vi "make magnet graph from elements.vi"(7 "mag type":enum16{"absolute", "relative", "positional"}(ring), 10 "toffset":dbl, 11 "elements":T2[](array[typedef])) -> (2 "t offset out":dbl, 3 "graphs":T1)   [LabVIEW 2017]
uses:
  typedefs/reading.ctl
  typedefs/readingType.ctl
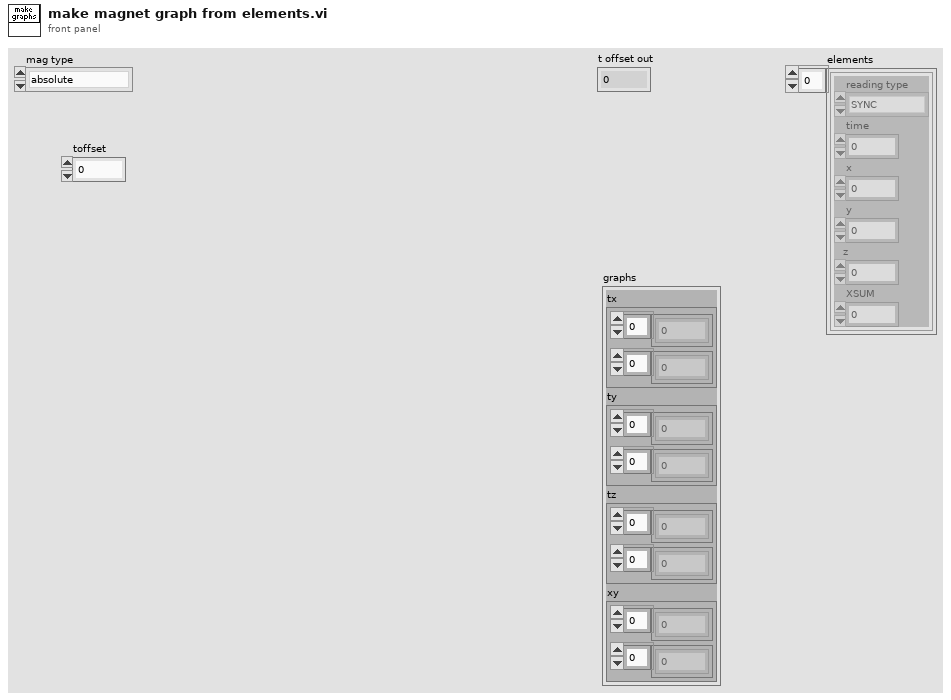
[diagram p1: front panel]
types:
  T1 = cluster{"tx":cluster{dbl[], sgl[]}, "ty":cluster{dbl[], sgl[]}, "tz":cluster{dbl[], sgl[]}, "xy":cluster{sgl[], sgl[]}}
  T2 = typedef "reading.ctl" = cluster{"reading type":T3, "time":fxp<+,48,48>, "x":sgl, "y":sgl, "z":sgl, "XSUM":u8}
  T3 = typedef "readingType.ctl" = enum8{"SYNC", "DETVAL", "COILI", "MAGVEC", "ACCVEC", "CROSSING", "MAGVEC0", "MAGVEC1", "MAGVEC2", "MAGVEC3", "MAGVEC4", "MAGVEC5", "MAGVEC6", "MAGVEC7"}
  T4 = cluster{"reading type":i32, "time":fxp<+,48,48>, "x":sgl, "y":sgl, "z":sgl, "XSUM":u8}
  T5 = cluster{"reading type":i32, "time":fxp<+,64,96>, "x":sgl, "y":sgl, "z":sgl, "XSUM":u8}
  T6 = cluster{"reading type":dbl, "time":dbl, "x":dbl, "y":dbl, "z":dbl, "XSUM":dbl}
  T7 = cluster{cluster{dbl[], sgl[]}, cluster{dbl[], sgl[]}, cluster{dbl[], sgl[]}, cluster{sgl[], sgl[]}}
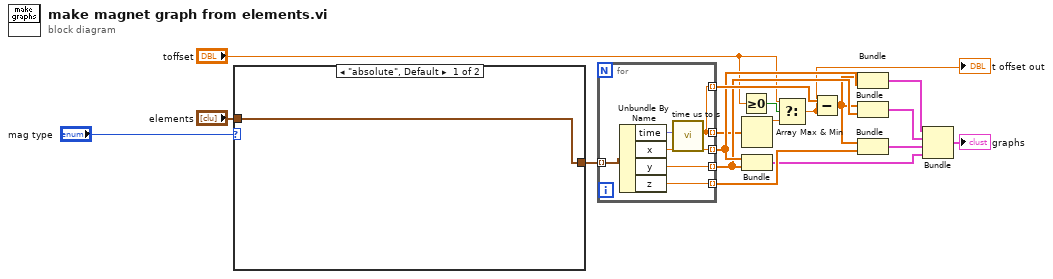
[diagram p0: block diagram]
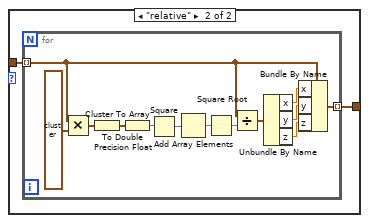
[diagram p2: hidden frame]
diagram:
  n1 = case shown="\"absolute\", Default" "mag type" {
    tunnel: "elements" -> [w19 w21]
    tunnel: [w19 w20] -> w2
    frame "absolute", Default {
    }
    frame "relative" {
      n2 = for {
        tunnel: w21 -> [w27] mode=indexing
        tunnel: [w22] -> w20 mode=indexing
        n3 = Multiply(x=w27, y=T4 {"reading type"=0, "time"=0.0, "x"=1.0, "y"=1.0, "z"=1.0, "XSUM"=0} ("reading3")) -> (x*y=w30:T5)
        n4 = To Double Precision Float(number=w30) -> (double precision float=w29:T6)
        n5 = Cluster To Array(cluster=w29) -> (array=w34:dbl[])
        n6 = Square(x=w34) -> (x^2=w33:dbl[])
        n7 = Add Array Elements(numeric array=w33) -> (sum=w32:dbl)
        n8 = Square Root(x=w32) -> (sqrt(x)=w31:dbl)
        n9 = Divide(x=w27, y=w31) -> (x/y=w26:T6)
        n10 = Unbundle By Name(w26) -> ("x"=w25:dbl, "y"=w24:dbl, "z"=w23:dbl)
        n11 = Bundle By Name(cluster=w27, "x"=w25, "y"=w24, "z"=w23) -> (w22:T2)
      }
    }
  }
  n12 = for {
    tunnel: w2 -> [w40] mode=indexing
    tunnel: [w35] -> w18 mode=indexing
    tunnel: [w39] -> w16 mode=indexing
    tunnel: [w38] -> w15 mode=indexing
    tunnel: [w37] -> w17 mode=indexing
    tunnel: [w35] -> w8 mode=indexing
    n13 = Unbundle By Name(w40) -> ("time"=w36:fxp<+,48,48>, "x"=w39:sgl, "y"=w38:sgl, "z"=w37:sgl)
    n14 = call "time us to s.vi"("time (us)"=w36) -> ("time (s)"=w35:dbl)  [unwired: 10 in]
  }
  n15 = Greater Or Equal To 0?(x="toffset") -> (x >= 0?=w7:bool)
  n16 = Array Max & Min(array=w8) -> (max value=w5:dbl)  [unwired: 3 out]
  n17 = Bundle(w16, w15) -> (w11:cluster{sgl[], sgl[]})  [unwired: 1 in]
  n18 = Select(t="toffset", s=w7, f=w5) -> (s? t:f=w4:dbl)
  "t offset out" <- w4
  n19 = Subtract(x=w18, y=w4) -> (x-y=w9:dbl[])
  n20 = Bundle(w9, w16) -> (w14:cluster{dbl[], sgl[]})  [unwired: 1 in]
  n21 = Bundle(w9, w15) -> (w13:cluster{dbl[], sgl[]})  [unwired: 1 in]
  n22 = Bundle(w9, w17) -> (w12:cluster{dbl[], sgl[]})  [unwired: 1 in]
  n23 = Bundle(w14, w13, w12, w11) -> (→"graphs":T7)  [unwired: 1 in]
